vi "Initialize Color Processors.vi"(8 "error in (no error)":errorcluster, 9 "Camera Color Correction Matrix":sgl[](array[numeric]), 10 "White Balance Matrix":sgl[](array[numeric]), 11 "BitDepth":i32) -> (0 "error out":errorcluster, 3 "Color Processor References":T1)   [LabVIEW 2015]
uses:
  C:/code/Host/Installer/Scientific Camera Interfaces/LabVIEW/32_bit/Library_X86/Thorlabs.TSI.Demosaicker.dll
  32_bit/Library_X86/Thorlabs.TSI.Demosaicker.dll
  C:/code/Host/Installer/Scientific Camera Interfaces/LabVIEW/32_bit/Library_X86/Thorlabs.TSI.ColorProcessor.dll
  32_bit/Library_X86/Thorlabs.TSI.ColorProcessor.dll
  C:/code/Host/Installer/Scientific Camera Interfaces/LabVIEW/32_bit/Library_X86/Thorlabs.TSI.ColorInterfaces.dll
  32_bit/Library_X86/Thorlabs.TSI.ColorInterfaces.dll
  Color/Color Processor References.ctl
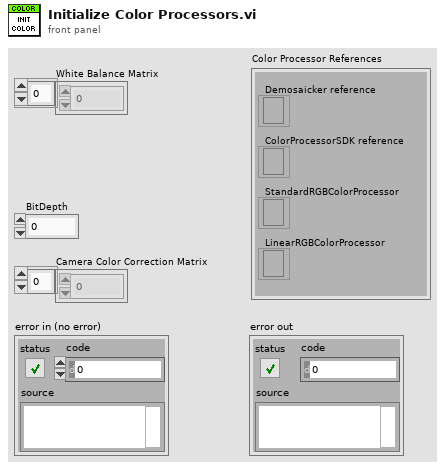
[diagram p1: front panel]
types:
  T1 = typedef "Color Processor References.ctl" = cluster{"Demosaicker reference":refnum<k24>, "ColorProcessorSDK reference":refnum<k24>, "StandardRGBColorProcessor":refnum<k24>, "LinearRGBColorProcessor":refnum<k24>}
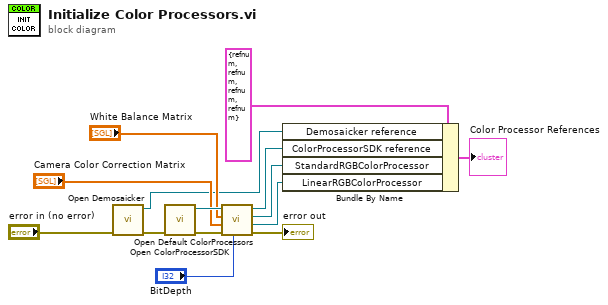
[diagram p0: block diagram]
diagram:
  n1 = call "Open Demosaicker.vi"("error in (no error)"="error in (no error)") -> ("error out"=w7:errorcluster, "Thorlabs.TSI.Demosaicker.Demosaicker"=w6:refnum<k24>)  [unwired: 9 in]
  n2 = call "Open ColorProcessorSDK.vi"("error in (no error)"=w7) -> ("error out"=w8:errorcluster, "Thorlabs.TSI.ColorProcessor.ColorProcessorSDK"=w12:refnum<k24>)  [unwired: 9 in]
  n3 = call "Open Default ColorProcessors.vi"("Bit Depth"="BitDepth", "error in (no error)"=w8, "Color Correction Matrix"="Camera Color Correction Matrix", "White Balance Matrix"="White Balance Matrix", "Thorlabs.TSI.ColorProcessor.ColorProcessorSDK"=w12) -> ("error out"=→"error out":errorcluster, 1:"Thorlabs.TSI.ColorInterfaces.IColorProcessor"=w3:refnum<k24>, 2:"Thorlabs.TSI.ColorInterfaces.IColorProcessor"=w4:refnum<k24>, "Thorlabs.TSI.ColorProcessor.ColorProcessorSDK"=w5:refnum<k24>)  [unwired: 3 in]
  n4 = Bundle By Name(cluster=T1 {"Demosaicker reference"=refnum, "ColorProcessorSDK reference"=refnum, "StandardRGBColorProcessor"=refnum, "LinearRGBColorProcessor"=refnum} ("Color Processor References"), "Demosaicker reference"=w6, "ColorProcessorSDK reference"=w5, "StandardRGBColorProcessor"=w4, "LinearRGBColorProcessor"=w3) -> (→"Color Processor References":T1)
